vi "PID_Control_Sim.vi"(1 "fc (Hz)":dbl=25.0, 2 "kp":dbl, 3 "y":dbl, 4 "r":dbl, 5 "kd":dbl, 6 "ki":dbl) -> (0 "u":dbl)   [LabVIEW 2011]
doc: "Proportional-integral-derivative (PID) controller implemented with the Simulation Module."
uses:
  <vilib>/Simulation/Implementation/Shared/SIMSCR Execution Mode.ctl
  <vilib>/Simulation/Scripting/Companion Diagram/SimConfigNode/SimParams.ctl
  <vilib>/Simulation/Scripting/Companion Diagram/SimConfigNode/_simSolvers.ctl
  <vilib>/Simulation/Param Hierarchy/Typedefs/SIMPH Param Control Actions.ctl
  <vilib>/Simulation/Implementation/Shared/SIM limit type.ctl
  <vilib>/Simulation/ContinuousLinear/Implementation/NILVSim Transfer Function Direct.llb/SIM Transfer Function Direct (SISO).vi
  <vilib>/Simulation/SignalArithmetic/Implementation/NILVSim Gain.llb/SIM Gain (scalar).vi
  <vilib>/Simulation/ContinuousLinear/Implementation/NILVSim Integrator new.llb/SIM Integrator distributor (scalar).vi
  <vilib>/Simulation/ContinuousLinear/Implementation/NILVSim Integrator new.llb/SIM Integrator collector (scalar).vi
  <vilib>/Simulation/Implementation/Shared/NILVSim_Manager.vi
  <vilib>/Simulation/Implementation/Shared/NILVSim_ParamChanged.vi
  <vilib>/Simulation/Implementation/Shared/NILVSim_FinalizeModel.vi
  <vilib>/Simulation/Implementation/Shared/SIM Unbundle Sim Info.vi
  <vilib>/Simulation/Implementation/Shared/NILVSim_GetModelError.vi
  <vilib>/Simulation/Implementation/Shared/SIM SimErrorHandler.vi
  <vilib>/Simulation/Implementation/Shared/SIM Bundle Sim Info.vi
  <vilib>/Simulation/Implementation/Shared/NILVSim_Initialize.vi
  <vilib>/Simulation/Scripting/Companion Diagram/SimConfigNode/SimDog.xnode
  <vilib>/Simulation/Implementation/XNodeFramework/SimXNode/SimX.xnode
  <vilib>/Simulation/ContinuousLinear/Implementation/NILVSim Integrator new.llb/SIM Integrator (scalar).vi
  <vilib>/Simulation/Implementation/Shared/NI_SIM_Implementation.lvlib
panel:
  in  "Transfer Function":cluster{"Numerator":dbl[], "Denominator":dbl[]}={"Numerator"=[1.0], "Denominator"=[1.0, 1.0]}
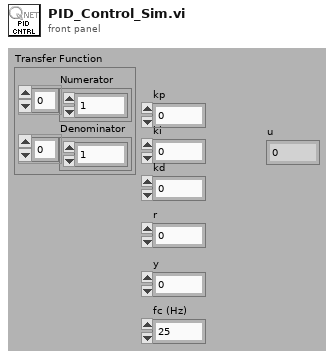
[diagram p1: front panel]
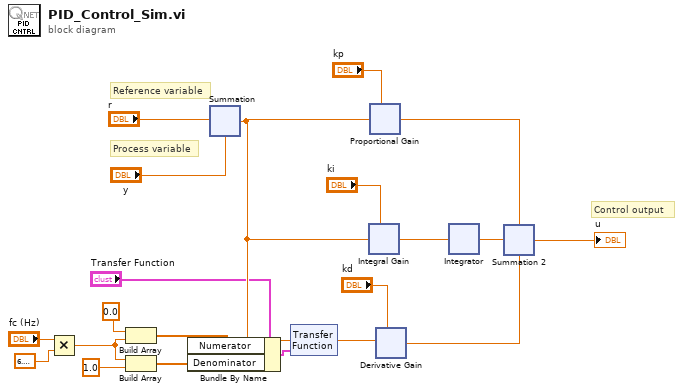
[diagram p0: block diagram]
diagram:
  # "Control output"
  # "Process variable"
  # "Reference variable"
  n1 = Multiply(x="fc (Hz)", y=6.283185307179586) -> (x*y=w1:dbl)
  n2 = Build Array(0.0, w1) -> (w6:dbl[])
  n3 = Build Array(w1, 1.0) -> (w5:dbl[])
  n4 = Bundle By Name(cluster="Transfer Function", "Numerator"=w6, "Denominator"=w5) -> (w4:cluster{"Numerator":dbl[], "Denominator":dbl[]})
  n5 = xnode ("Summation")("Operand1"="r", "Operand2"="y") -> ("Result"=w9:dbl)
  n6 = xnode ("Transfer Function")("input u(k)"=w9, "Transfer Function"=w4) -> ("output y(k)"=w8:dbl)  [unwired: 3 in, 1 out]
  n7 = xnode "Integral Gain"("gain"="ki", "input"=w9) -> ("output"=w16:dbl)  [unwired: 2 in]
  n8 = xnode "Proportional Gain"("gain"="kp", "input"=w9) -> ("output"=w18:dbl)  [unwired: 2 in]
  n9 = xnode "Derivative Gain"("gain"="kd", "input"=w8) -> ("output"=w13:dbl)  [unwired: 2 in]
  n10 = xnode ("Integrator")("input"=w16) -> ("output"=w14:dbl)  [unwired: 9 in, 2 out]
  n11 = xnode ("Summation 2")("Operand1"=w18, "Operand2"=w14, "Operand3"=w13) -> ("Result"=→"u":dbl)
